vi "Translator.Init.vi"(8 "error in":errorcluster, 10 "Language in":string, 11 "Translation folder":path=path "D:/PL_0125_Sapphire_Automation/settings") -> (0 "error out":errorcluster, 2 "Language out":string)   [LabVIEW 2016]
uses:
  Translator.Enums.ctl
  Translator.Message.ctl
  EventLog/EventLog.EventLevelGui.ctl
  Windows/Windows.ExitAction.ctl
  TouchPanel/TouchPanelMonths.ctl
  EventLog/EventLog.EventSource.ctl
  Translator.Control.Fglb.Action.vi
  Translator.Global.vi
panel:
  in  "Enums":T1={"Msg"=enum."Quitting", "Level"=enum."ALL", "ExitAction"=enum."Log off from PC", "Month"=enum."January", "Source"=enum."Gui"}
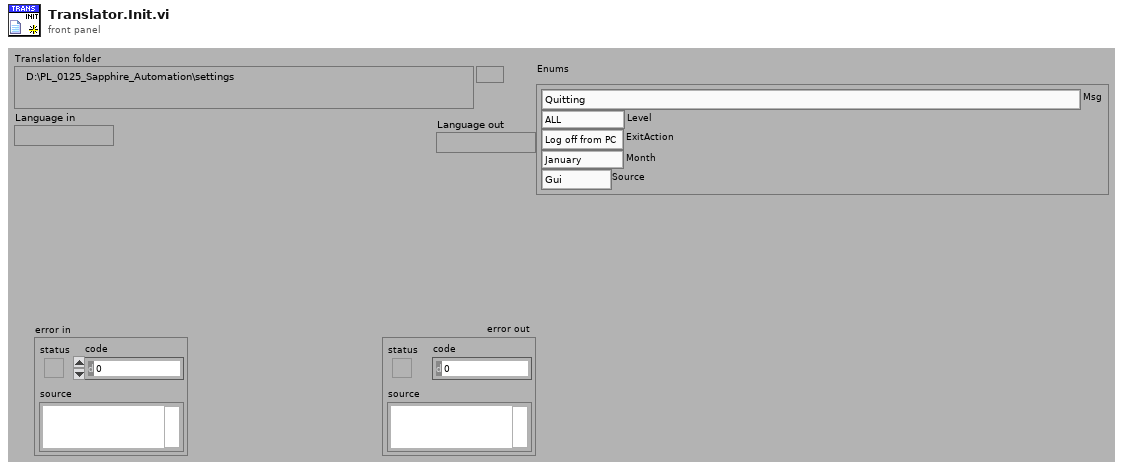
[diagram p1: front panel]
types:
  T1 = typedef "Translator.Enums.ctl" = cluster{"Msg":T2, "Level":T3, "ExitAction":T4, "Month":T5, "Source":T6}
  T2 = typedef "Translator.Message.ctl" = enum16{"-", "Event confirmed", "Log out", "Log in", "Shutdown", "Cancel", "Start", "Continue", "Stop", "On", "Off", "OK", "NOK", "NOK %s", "This", "Prev", "Home", "Work", "In progress...", "Missing", "Empty", "Hardware failure", "Initial", "Error %d >> %s", "Error %d >> %s >> %s", "Starting %s", "Quitting %s", "Configured", "Initializing", "Quitting", "Loading", "Running %s", "Stopped", "Summary", "Do you want to continue?", "Do you want to exit?", "Log out?", "System", "All", "IDLE", "Translating...%s", "Not found", "Alarm %s", "Run", "Skip", "Abort", "Repeat", "Please wait...", "Database disconnected", "Login to database successful", "Login to database failed: %d; %s", "Get process step data for %s", "Changeover off", "Changeover into %s", "Product %s | %s found in cache with status %d at previous station", "Product %s | %s found in database with status %d at previous station", "Product %s | %s not found in cache at previous station", "Product %s | %s not found in database at previous station", "Product %s | %s found in cache with status %d at this station (%d repetion)", "Product %s | %s found in database with status %d at this station (%d repetition)", "Product %s | %s not found in cache at this station", "Product %s | %s not found in database at this station", "Product %s | %s found in cache for component %s | %s", "Product %s | %s found in database for component %s | %s", "Product not found in cache for component %s | %s", "Product not found in database for component %s | %s", "Product %s | %s connected with component %s | %s (cache)", "Product %s | %s connected with component %s | %s (database)", "New data for %s | %s (cache)", "New data for %s | %s (database)", "File %s moved (cache)", "File %s deleted (cache)", "Msg %d >> %s", "PLC LifeBit Failure", "Reconnecting DB", "Reconnecting PLC", "Free disk space is below 1GB - contact technician", "Unable to check product status", "Product %s SN %s checked in DB", "Unable To check status from station %s"}
  T3 = typedef "EventLog.EventLevelGui.ctl" = enum16{"ALL", "Debug", "Info", "Warning", "Error"}
  T4 = typedef "Windows.ExitAction.ctl" = enum16{"Log off from PC", "Shut Down PC", "Reboot PC", "Close Program"}
  T5 = typedef "TouchPanelMonths.ctl" = enum16{"January", "February", "March", "April", "May", "June", "July", "August", "September", "October", "November", "December"}
  T6 = typedef "EventLog.EventSource.ctl" = enum16{"All", "Gui", "Cache", "PLC1", "PLC2", "PLC3", "DB", "DB01", "DB02", "DB03", "DB04", "DB05", "DB06", "DB07", "DB08", "DB09", "DB10", "DB11", "DB12", "DB13", "DB14", "DB15", "DB16"}
  T7 = typedef "Translator.Control.Fglb.Action.vi" = enum16{"init", "set", "get", "clear"}
  T8 = enum32{"invalid app kind", "Development System", "Run Time System", "Student Edition", "Embedded LabVIEW", "Evaluation", "Custom"}
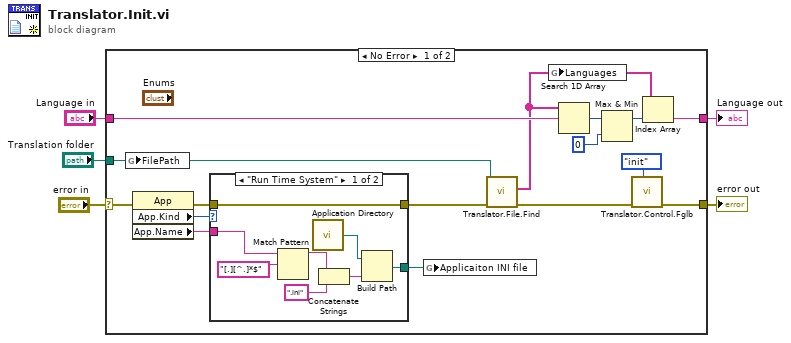
[diagram p0: block diagram]
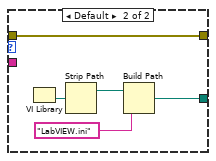
[diagram p2: hidden frame]
diagram:
  n1 = case shown="No Error" "error in" {
    selector: "error in" -> [w19 w36]
    tunnel: [w8 w36] -> w5
    tunnel: "Translation folder" -> [w6 _]
    tunnel: "Language in" -> [w13 w35]
    tunnel: [w11 w35] -> w1
    frame No Error {
      n2 = global write "Translator.Global.vi" "FilePath"(w6) -> ()
      n3 = property class="App"(error in=w19) -> (error out=w21:errorcluster, "App.Kind"=w20:T8, "App.Name"=w10:string)  [unwired: 1 in, 1 out]
      n4 = case shown="\"Run Time System\"" w20 {
        tunnel: [w29 w34] -> w18
        tunnel: w21 -> [w29 w34]
        tunnel: [w27 w30] -> w14
        tunnel: w10 -> [w25 _]
        frame "Run Time System" {
          n5 = Match Pattern(string=w25, regular expression="[.][^.]*$") -> (before substring=w24:string)  [unwired: 4 out]
          n6 = call <vilib>:"Application Directory.vi"() -> ("Application Directory"=w28:path)
          n7 = Concatenate Strings(w24, ".ini" ("string")) -> (w22:string)
          n8 = Build Path(base path=w28, name or relative path=w22) -> (appended path=w27:path)
        }
        frame Default {
          n9 = VI Library() -> (path=w33:path)
          n10 = Strip Path(path=w33) -> (stripped path=w32:path)  [unwired: 1 out]
          n11 = Build Path(base path=w32, name or relative path="LabVIEW.ini") -> (appended path=w30:path)
        }
      }
      n12 = global write "Translator.Global.vi" "Applicaiton INI file"(w14) -> ()
      n13 = call "Translator.File.Find.vi"("error in"=w18, "Translation folder"=w6) -> ("error out"=w9:errorcluster, "Languages"=w12:string[])  [unwired: 8 in]
      n14 = global write "Translator.Global.vi" "Languages"(w12) -> ()
      n15 = Search 1D Array(1D array=w12, element=w13) -> (index of element=w15:i32)  [unwired: 1 in]
      n16 = Max & Min(x=w15, y=0) -> (max(x,y)=w16:i32)  [unwired: 1 out]
      n17 = call "Translator.Control.Fglb.vi"("Action"=Translator.Control.Fglb.Action.vi."init", "error in (no error)"=w9) -> ("error out"=w8:errorcluster)  [unwired: 8 in, 1 out]
      n18 = Index Array(array=w12, index=w16) -> (element=w11:string)
    }
    frame Error {
    }
  }
  "error out" <- w5
  "Language out" <- w1
